vi "Enable Disable Routing Channel.vi"(8 "error in (no error)":errorcluster, 11 "Node Ptr":u64 format="%.0x") -> (0 "error out":errorcluster, 3 "Node Ptr out":T1 format="%.0x")   [LabVIEW 2020, in "Routing and Faulting System Explorer.lvlib"]
uses:
  Routing and Faulting System Explorer.lvlib
  <vilib>/NI VeriStand/Custom Device API/Custom Device Item Ref.ctl
  Shared/Constants.vi
  <vilib>/NI VeriStand/Custom Device API/Custom Device API.lvlib
  Shared/Routing and Faulting Shared.lvlib
  Scripting/Routing and Faulting Scripting.lvlib
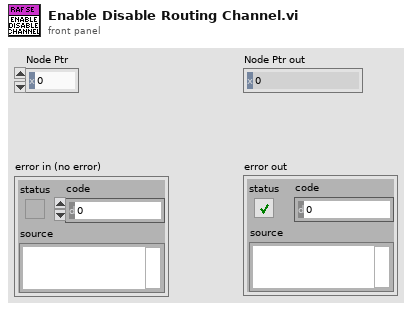
[diagram p1: front panel]
types:
  T1 = typedef "Custom Device API.lvlib/Custom Device Item Ref.ctl" = u64
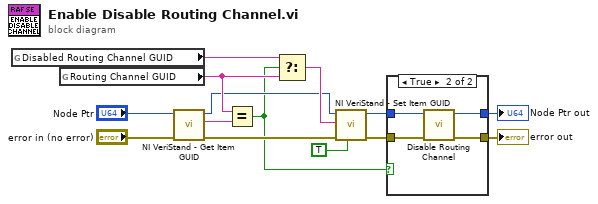
[diagram p0: block diagram]
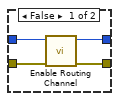
[diagram p2: hidden frame]
diagram:
  n1 = global read "Constants.vi" "Disabled Routing Channel GUID"() -> (w11:string)
  n2 = global read "Constants.vi" "Routing Channel GUID"() -> (w10:string)
  n3 = call <vilib>:"NI VeriStand - Get Item GUID.vi"("error in (no error)"="error in (no error)", "Item Ref in"="Node Ptr") -> ("error out"=w9:errorcluster, "GUID"=w12:string, "Item Ref out"=w7:T1)  [unwired: 7 in]
  n4 = Equal?(x=w10, y=w12) -> (x = y?=w5:bool)
  n5 = Select(t=w11, s=w5, f=w10) -> (s? t:f=w8:string)
  n6 = call <vilib>:"NI VeriStand - Set Item GUID.vi"("Refresh System Explorer Tree? (F)"=TRUE, "error in (no error)"=w9, "GUID"=w8, "Item Ref in"=w7) -> ("error out"=w4:errorcluster, "Item Ref out"=w3:T1)  [unwired: 6 in]
  n7 = case shown="True" w5 {
    tunnel: w4 -> [w18 w22]
    tunnel: w3 -> [w17 w21]
    tunnel: [w16 w20] -> w2
    tunnel: [w15 w19] -> w1
    frame False {
      n8 = call "Enable Routing Channel.vi"("error in"=w18, "routing channel in"=w17) -> ("error out"=w15:errorcluster, "routing channel out"=w16:T1)  [unwired: 8 in]
    }
    frame True {
      n9 = call "Disable Routing Channel.vi"("error in"=w22, "routing channel in"=w21) -> ("error out"=w19:errorcluster, "routing channel out"=w20:T1)  [unwired: 8 in]
    }
  }
  "Node Ptr out" <- w2
  "error out" <- w1
